vi "CheckPlane.vi"(1 "plane 2":u32) -> (0 "plane":u32)   [LabVIEW 2009]
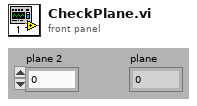
[diagram p1: front panel]
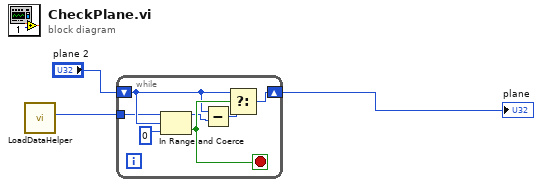
[diagram p0: block diagram]
diagram:
  n1 = call "LoadDataHelper.vi"() -> ("planes"=w1:u32)  [unwired: 7 in, 4 out]
  n2 = while {
    tunnel: w1 -> [w5]
    shift-right: [w7] -> w3
    shift-left: "plane 2" -> [w6]
    stop <- w8 stop-if-true
    n3 = In Range and Coerce(upper limit=w5, x=w6, lower limit=u32 0) -> (In Range?=w8:bool)  [unwired: 1 out]
    n4 = Subtract(x=w6, y=w5) -> (x-y=w4:u32)
    n5 = Select(t=w6, s=w8, f=w4) -> (s? t:f=w7:u32)
  }
  "plane" <- w3
